vi "Untitled 3.vi"() -> ()   [LabVIEW 2014]
uses:
  AD4212C.lvlib
panel:
  out "error out":errorcluster
  out "Weight":dbl format="%.2f"
  in  "VISA resource name":refnum<visa-resource-name>="COM1"
  in  "Serial Configuration":T1={"Baud Rate (2400)"=2400, "Flow Control (0: None)"=0, "Parity (2: Even)"=2, "Data Bits (7)"=7} {"Data Bits (7)" items=["7"=7, "8"=8]; "Parity (2: Even)" items=["None", "Odd", "Even"]; "Flow Control (0: None)" items=["None"=0, "RTS/CTS"=2]; "Baud Rate (2400)" items=["600"=600, "1200"=1200, "2400"=2400, "4800"=4800, "9600"=9600, "19200"=19200]}
  in  "error in (no error)":errorcluster
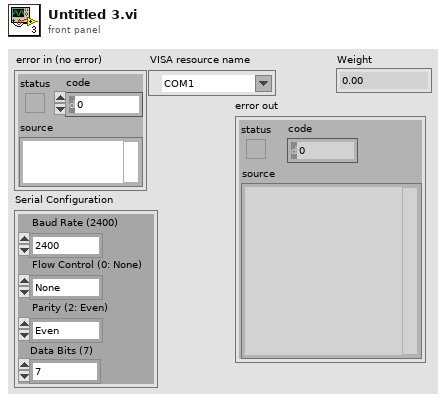
[diagram p1: front panel]
types:
  T1 = cluster{"Baud Rate (2400)":u32, "Flow Control (0: None)":u16, "Parity (2: Even)":u16, "Data Bits (7)":u16}
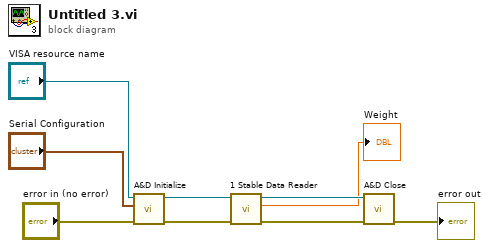
[diagram p0: block diagram]
diagram:
  n1 = call "A&D Initialize.vi"("error in (no error)"="error in (no error)", "Serial Configuration"="Serial Configuration", "VISA resource name"="VISA resource name") -> ("error out"=w6:errorcluster, "VISA resource name out"=w9:refnum<visa-resource-name>)  [unwired: 7 in]
  n2 = call "1 Stable Data Reader.vi"("error in"=w6, "VISA resource name"=w9) -> ("error out"=w7:errorcluster, "Weight"=→"Weight":dbl, "VISA resource name out"=w8:refnum<visa-resource-name>)  [unwired: 6 in, 1 out]
  n3 = call "A&D Close.vi"("error in (no error)"=w7, "VISA resource name"=w8) -> ("error out"=→"error out":errorcluster)  [unwired: 9 in]
